vi "PWM Input Post Step.vi"(8 "error in (no error)":errorcluster, 9 "PWM Input In":T1, 10 "Socket No":u16=1, 11 "PWM Input in":refnum<class "PWM Input.lvclass">) -> (0 "error out":errorcluster, 1 "AnalogRead":dbl[](array[numeric]), 2 "Report Text":string, 3 "PWM Input out":refnum<class "PWM Input.lvclass">, 4 "Duty Cycle":dbl[](array[numeric]), 5 "Physical Channel":string[](array[string]))   [LabVIEW 2023, in "HardwareAbstractionLayer_LVOOP.lvlib" / "PWM Input.lvclass"]
uses:
  PWM Input.lvclass
  NI PWM Input_class/NI PWM DAQ/Control/PWMInputEdit.ctl
  NI PWM Input_class/NI PWM Input.lvclass
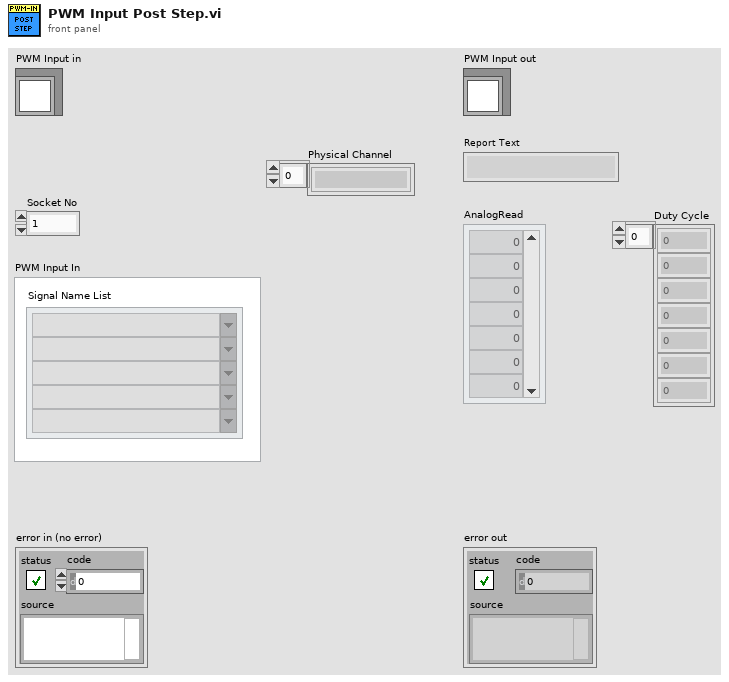
[diagram p1: front panel]
types:
  T1 = typedef "HardwareAbstractionLayer_LVOOP.lvlib/NI PWM Input.lvclass/PWMInputEdit.ctl" = cluster{"Signal Name List":string[]}
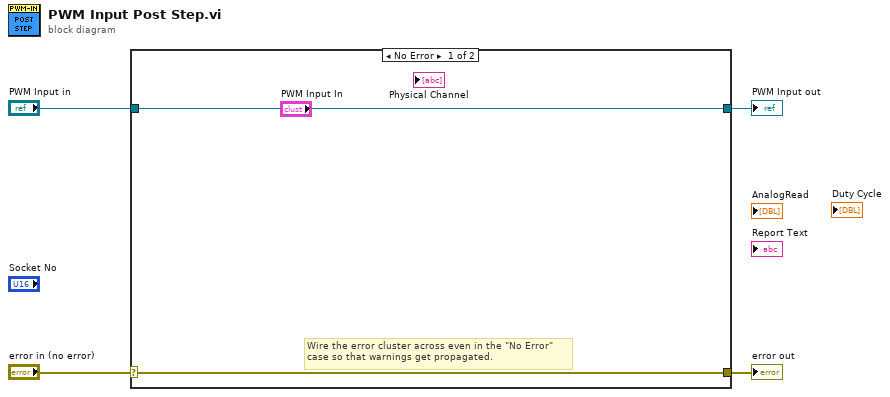
[diagram p0: block diagram]
diagram:
  n1 = case shown="No Error" "error in (no error)" {
    selector: "error in (no error)" -> [w5 w8]
    tunnel: [w5 w8] -> w3
    tunnel: [w6 w7] -> w1
    tunnel: "PWM Input in" -> [w6 w7]
    frame No Error {
      # "Wire the error cluster across even in the \"No Error\"\ncase so that warnings get propagated."
    }
    frame Error {
    }
  }
  "error out" <- w3
  "PWM Input out" <- w1
